vi "Save Accel math.vi"(4 "Final Accel Values":dbl[][](array[numeric]), 5 "Final Accel Values 1":dbl[][](array[numeric]), 6 "Final Accel Values 2":dbl[][](array[numeric]), 7 "Final Accel Values 3":dbl[][](array[numeric]), 8 "Final Accel Values 4":dbl[][](array[numeric]), 9 "Final Accel Values 5":dbl[][](array[numeric]), 10 "Base Accels":dbl[][](array[numeric]), 11 "Six Plane Accels":dbl[][](array[numeric])) -> ()   [LabVIEW 2013]
uses:
  <vilib>/Utility/NIReport.llb/NI_report.lvclass
  <vilib>/addons/_office/NI_ReportGenerationToolkit.lvlib
  <vilib>/addons/_office/excel.llb/Excel Easy Table (num).vi
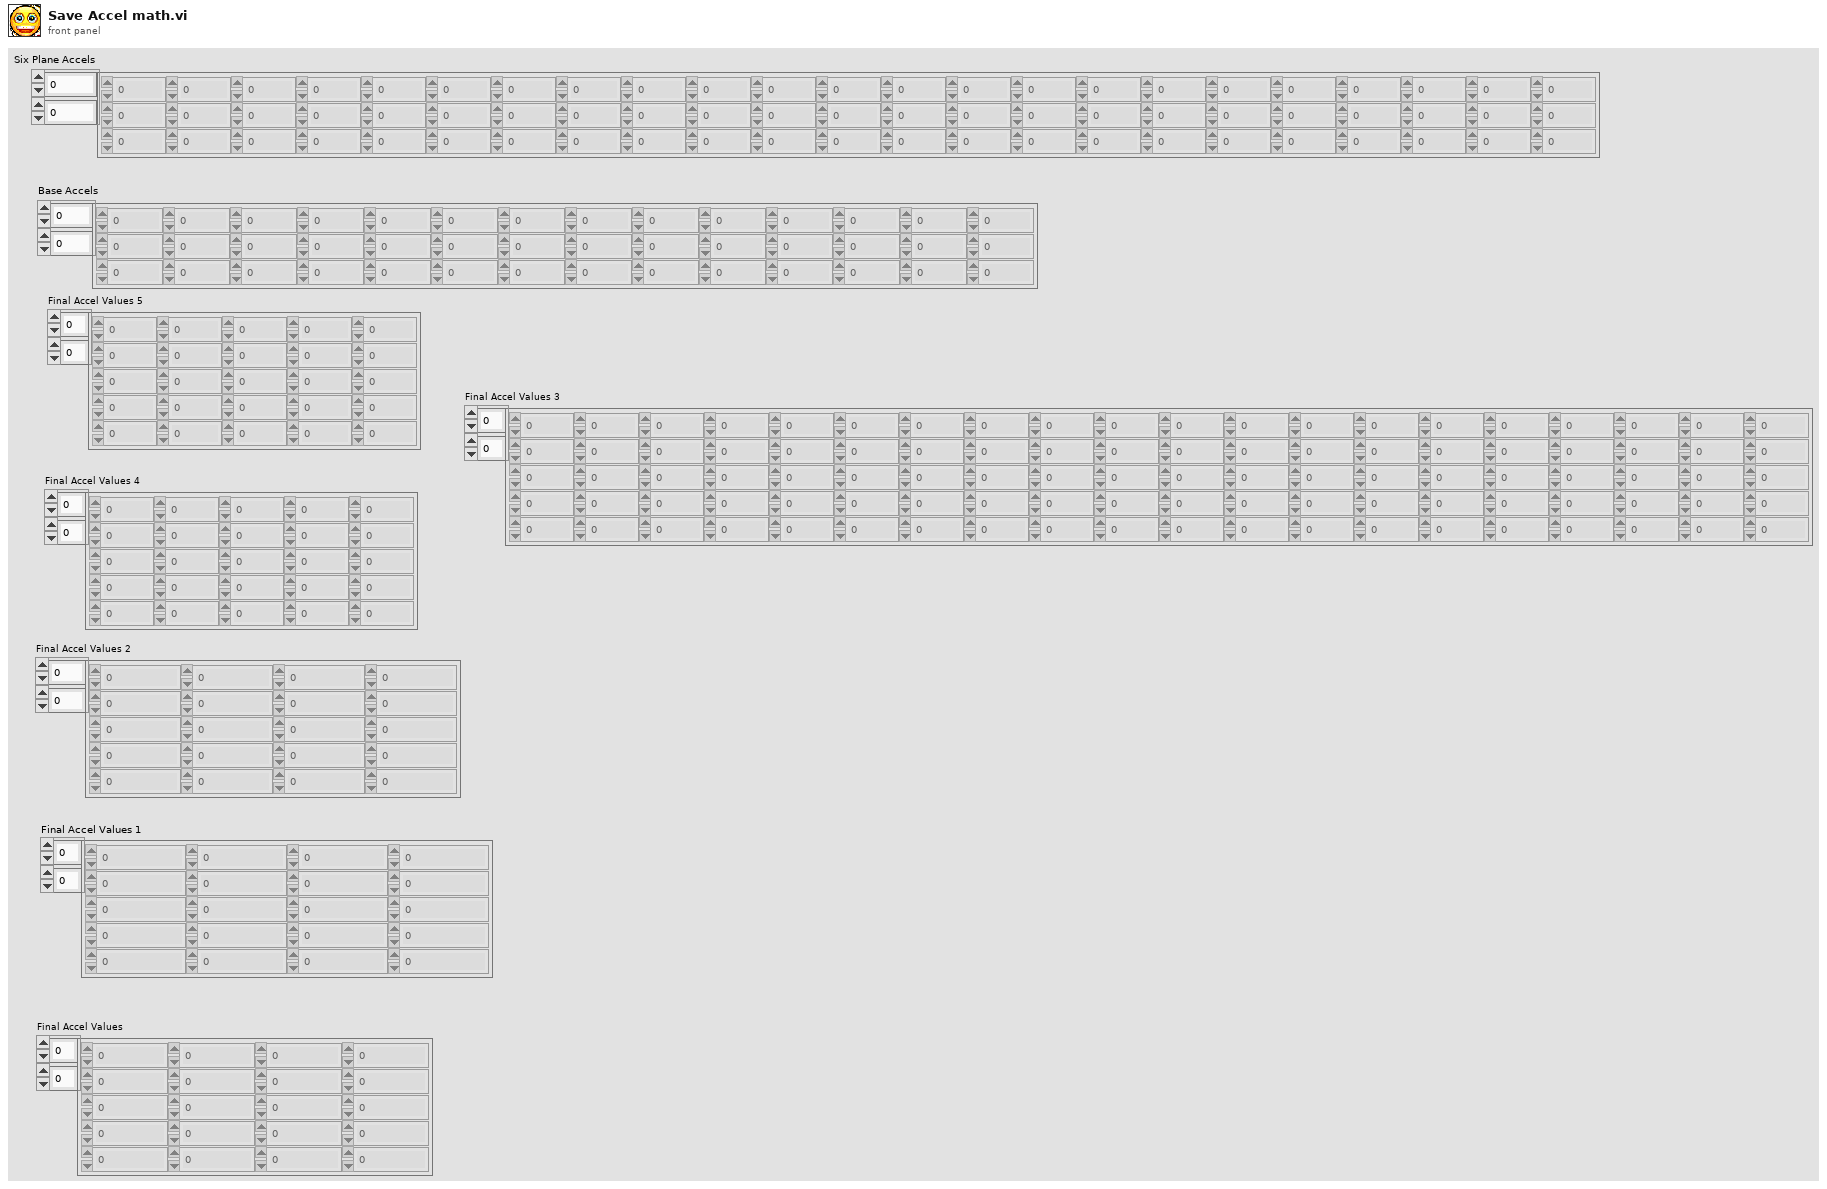
[diagram p1: front panel]
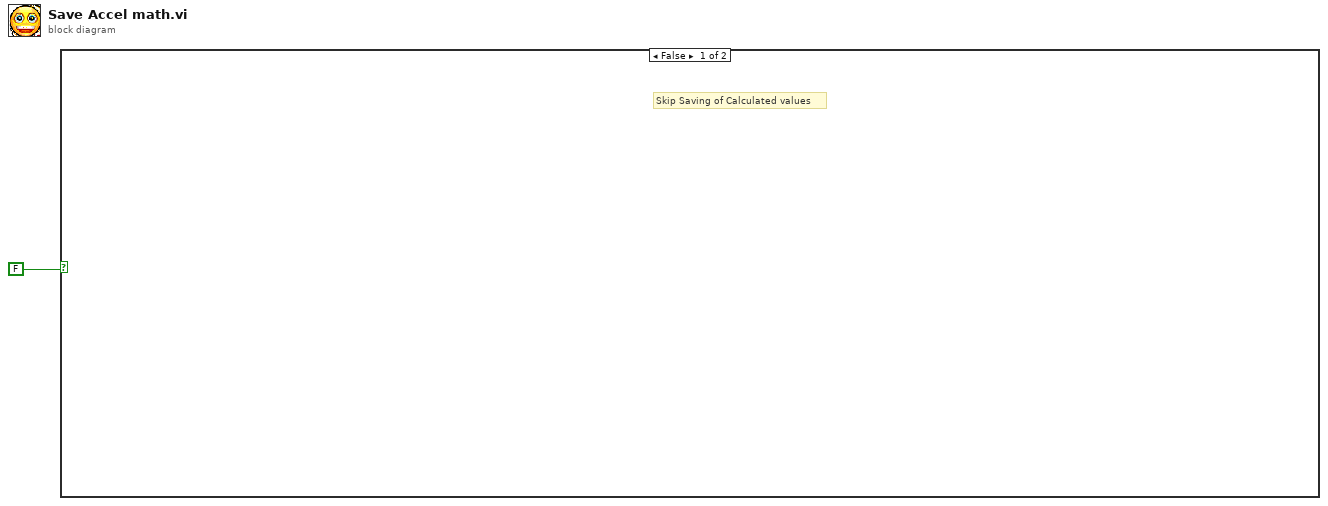
[diagram p0: block diagram]
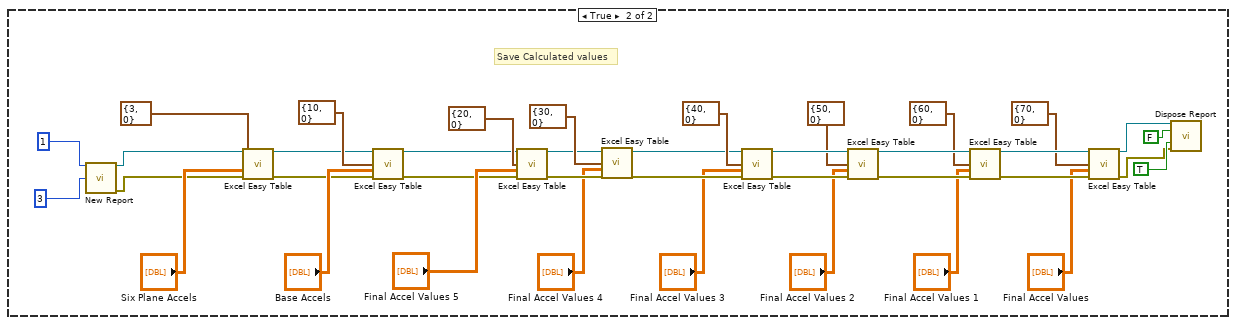
[diagram p2: hidden frame]
diagram:
  n1 = case shown="False" FALSE {
    frame False {
      # "Skip Saving of Calculated values"
    }
    frame True {
      # "Save Calculated values"
      n2 = call <vilib>:"New Report.vi"("window state (normal)"=1, "report type"=3) -> ("report out"=w14:refnum<class "NI_report.lvclass">, "error out"=w13:errorcluster)  [unwired: 12 in]
      n3 = call-poly <vilib>:"Excel Easy Table.vi"("report in"=w14, "start (0, 0)"=cluster{"row":i32, "column":i32} {"row"=3, "column"=0} ("start (-1, -1)"), "text data"="Six Plane Accels", "error in (no error)"=w13) -> ("report out"=w16:refnum<class "NI_report.lvclass">, "error out"=w15:errorcluster)  [unwired: 7 in, 3 out]
      n4 = call-poly <vilib>:"Excel Easy Table.vi"("report in"=w16, "start (0, 0)"=cluster{"row":i32, "column":i32} {"row"=10, "column"=0} ("start (-1, -1)"), "text data"="Base Accels", "error in (no error)"=w15) -> ("report out"=w18:refnum<class "NI_report.lvclass">, "error out"=w17:errorcluster)  [unwired: 7 in, 3 out]
      n5 = call-poly <vilib>:"Excel Easy Table.vi"("report in"=w18, "start (0, 0)"=cluster{"row":i32, "column":i32} {"row"=20, "column"=0} ("start (-1, -1)"), "text data"="Final Accel Values 5", "error in (no error)"=w17) -> ("report out"=w4:refnum<class "NI_report.lvclass">, "error out"=w5:errorcluster)  [unwired: 7 in, 3 out]
      n6 = call-poly <vilib>:"Excel Easy Table.vi"("report in"=w4, "start (0, 0)"=cluster{"row":i32, "column":i32} {"row"=30, "column"=0} ("start (-1, -1)"), "text data"="Final Accel Values 4", "error in (no error)"=w5) -> ("report out"=w8:refnum<class "NI_report.lvclass">, "error out"=w7:errorcluster)  [unwired: 7 in, 3 out]
      n7 = call-poly <vilib>:"Excel Easy Table.vi"("report in"=w8, "start (0, 0)"=cluster{"row":i32, "column":i32} {"row"=40, "column"=0} ("start (-1, -1)"), "text data"="Final Accel Values 3", "error in (no error)"=w7) -> ("report out"=w37:refnum<class "NI_report.lvclass">, "error out"=w34:errorcluster)  [unwired: 7 in, 3 out]
      n8 = call-poly <vilib>:"Excel Easy Table.vi"("report in"=w37, "start (0, 0)"=cluster{"row":i32, "column":i32} {"row"=50, "column"=0} ("start (-1, -1)"), "text data"="Final Accel Values 2", "error in (no error)"=w34) -> ("report out"=w36:refnum<class "NI_report.lvclass">, "error out"=w33:errorcluster)  [unwired: 7 in, 3 out]
      n9 = call-poly <vilib>:"Excel Easy Table.vi"("report in"=w36, "start (0, 0)"=cluster{"row":i32, "column":i32} {"row"=60, "column"=0} ("start (-1, -1)"), "text data"="Final Accel Values 1", "error in (no error)"=w33) -> ("report out"=w35:refnum<class "NI_report.lvclass">, "error out"=w32:errorcluster)  [unwired: 7 in, 3 out]
      n10 = call-poly <vilib>:"Excel Easy Table.vi"("report in"=w35, "start (0, 0)"=cluster{"row":i32, "column":i32} {"row"=70, "column"=0} ("start (-1, -1)"), "text data"="Final Accel Values", "error in (no error)"=w32) -> ("report out"=w10:refnum<class "NI_report.lvclass">, "error out"=w9:errorcluster)  [unwired: 7 in, 3 out]
      n11 = call-dynamic "Dispose Report.vi"("report in"=w10, "wait until printing completed? (T)"=FALSE, "save changes? (F)"=TRUE, "error in (no error)"=w9) -> ()  [unwired: 11 in, 1 out]
    }
  }
